vi "AddToChartCollection.vi"(0 "reference in":refnum<class "LcWebView.lvclass">, 1 "Chart Content":T1, 5 "error in (no error)":errorcluster) -> (14 "reference out":refnum<class "LcWebView.lvclass">, 19 "error out":errorcluster)   [LabVIEW 2018, in "LcWebView.lvclass"]
uses:
  LcWebView.lvclass
  ctrls/ChartContent.ctl
  ctrls/ChartSetup.ctl
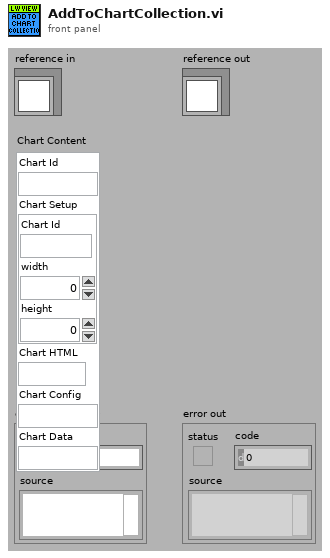
[diagram p1: front panel]
types:
  T1 = typedef "LcWebView.lvclass/ChartContent.ctl" = cluster{"Chart Id":string, "Chart Setup":T2, "Chart HTML":string, "Chart Config":string, "Chart Data":string}
  T2 = typedef "LcWebView.lvclass/ChartSetup.ctl" = cluster{"Chart Id":string, "width":u32, "height":u32}
  T3 = typedef "LcWebView.lvclass/ObjectAttributes.ctl" = cluster{"WebView Container":refnum<k24>, "CoreWebViewRef":refnum<k24>, "Status":i32, "Status Message":string, "User Data Folder":path, "BrowserProcessId":u32, "PlotType":T4, "Chart Collection":T5}
  T4 = typedef "LcWebView.lvclass/PlotType.ctl" = enum16{"bar", "line", "pie"}
  T5 = typedef "LcWebView.lvclass/ChartCollection.ctl" = T1[]
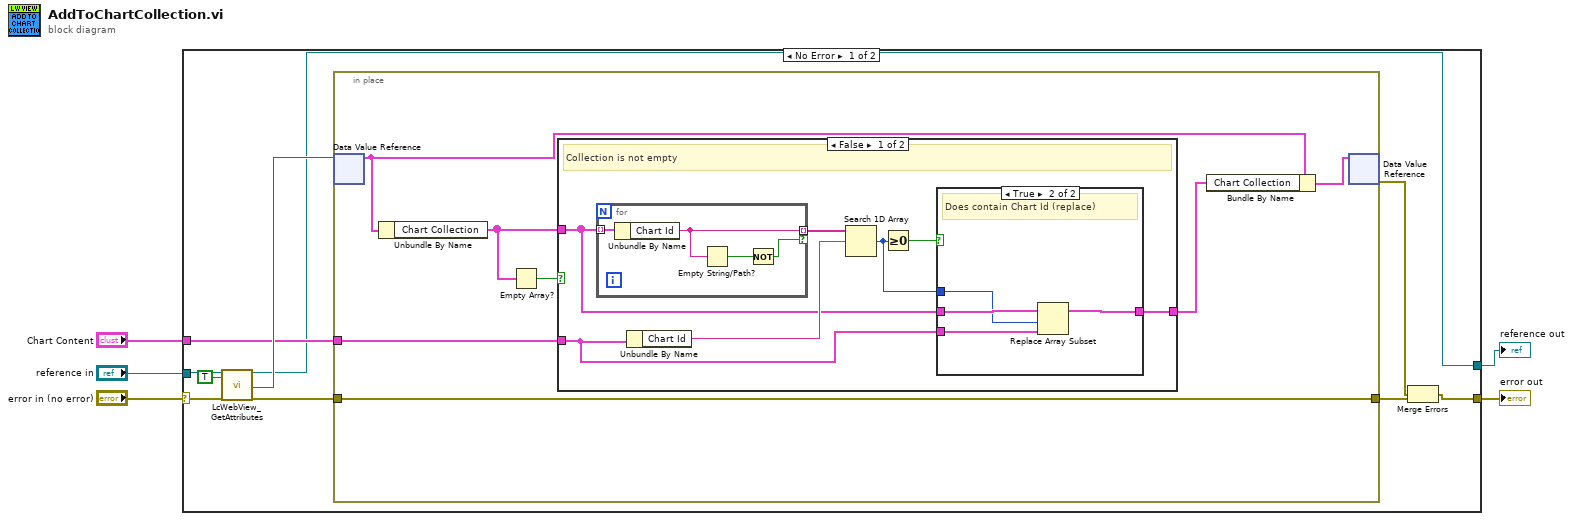
[diagram p0: block diagram]
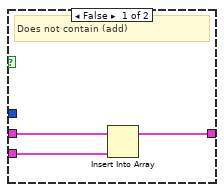
[diagram p2: hidden frame]
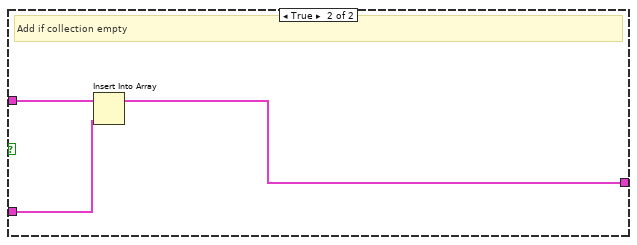
[diagram p3: hidden frame]
diagram:
  n1 = case shown="No Error" "error in (no error)" {
    selector: "error in (no error)" -> [w15 w45]
    tunnel: [w6 w45] -> w4
    tunnel: [w9 w44] -> w2
    tunnel: "reference in" -> [w14 w44]
    tunnel: "Chart Content" -> [w10 _]
    frame No Error {
      n2 = call "LcWebView_GetAttributes.vi"("reference in"=w14, "OnlyGetDvrReference(False)"=TRUE, "error in (no error)"=w15) -> ("reference out"=w9:refnum<class "LcWebView.lvclass">, "DataRef"=w13:refnum<data-value>, "error out"=w11:errorcluster)  [unwired: 13 in, 1 out]
      n3 = in-place {
        in-place-border: w11 -> [w16]
        in-place-border: w10 -> [w20]
        in-place-border: [w16] -> w8
        n4 = in-place-dvr #1(w13) -> (w19:T3)  [unwired: 1 out]
        n5 = Unbundle By Name(w19) -> ("Chart Collection"=w21:T5)
        n6 = Empty Array?(array=w21) -> (empty?=w22:bool)
        n7 = case shown="False" w22 {
          tunnel: w21 -> [w26 w43]
          tunnel: w20 -> [w25 w42]
          tunnel: [w24 w41] -> w18
          frame False {
            # "Collection is not empty"
            n8 = for {
              tunnel: w26 -> [w40] mode=indexing
              tunnel: [w39] -> w29 mode=indexing if=w37
              n9 = Unbundle By Name(w40) -> ("Chart Id"=w39:string)
              n10 = Empty String/Path?(string/path=w39) -> (empty?=w38:bool)
              n11 = Not(x=w38) -> (.not. x?=w37:bool)
            }
            n12 = Unbundle By Name(w25) -> ("Chart Id"=w28:string)
            n13 = Search 1D Array(1D array=w29, element=w28) -> (index of element=w23:i32)  [unwired: 1 in]
            n14 = Greater Or Equal To 0?(x=w23) -> (x >= 0?=w27:bool)
            n15 = case shown="True" w27 {
              tunnel: w26 -> [w32 w36]
              tunnel: w25 -> [w31 w34]
              tunnel: [w30 w33] -> w24
              tunnel: w23 -> [_ w35]
              frame False {
                # "Does not contain (add)"
                n16 = Insert Into Array(array=w32, new element=w31) -> (w30:T5)  [unwired: 1 in]
              }
              frame True {
                # "Does contain Chart Id (replace)"
                n17 = Replace Array Subset(array=w36, new element=w34, index=w35) -> (w33:T5)
              }
            }
          }
          frame True {
            # "Add if collection empty"
            n18 = Insert Into Array(array=w43, new element=w42) -> (w41:T5)  [unwired: 1 in]
          }
        }
        n19 = Bundle By Name(cluster=w19, "Chart Collection"=w18) -> (w17:T3)
        n20 = in-place-dvr #1(w17) -> (w7:errorcluster)  [unwired: 1 out]
      }
      n21 = Merge Errors(w7, w8) -> (w6:errorcluster)
    }
    frame Error {
    }
  }
  "error out" <- w4
  "reference out" <- w2
